vi "GetMemeoryUsagePC.vi"() -> (0 "Fehler (Ausgang)":errorcluster, 1 "largest contiguous (bytes)":dbl, 2 "available (bytes)":dbl, 3 "total (bytes)":dbl)   [LabVIEW 2020, in "Erweiterte Konfig.lvlib" / "System Load.lvlib"]
uses:
  <vilib>/nisyscfg/Close (System).vi
  System Load.lvlib
  <vilib>/nisyscfg/nisyscfg.lvlib
  <resource>/objmgr/nisysapi.rc
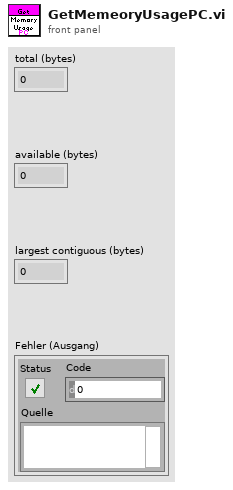
[diagram p1: front panel]
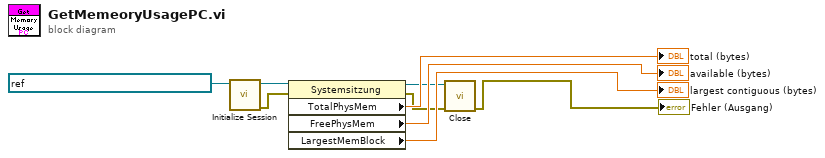
[diagram p0: block diagram]
diagram:
  n1 = call <vilib>:"Initialize Session.vi"("Target (localhost)"=refnum<k21> "NI-cRIO-9066-IAG (192.168.14.14)") -> ("error out"=w4:errorcluster, "Session out"=w3:refnum<k21>)  [unwired: 9 in]
  n2 = property class="Systemsitzung"(reference=w3, error in=w4) -> (reference out=w2:refnum<k21>, error out=w1:errorcluster, "TotalPhysMem"=→"total (bytes)":dbl, "FreePhysMem"=→"available (bytes)":dbl, "LargestMemBlock"=→"largest contiguous (bytes)":dbl)
  n3 = call-poly <vilib>:"Close.vi"("error in (no error)"=w1, "Session in"=w2) -> ("error out"=→"Fehler (Ausgang)":errorcluster)  [unwired: 9 in]
